vi "Set Quality Check Observables.vi"(8 "error in (no error)":errorcluster, 10 "Obsv to check":T1(array[cluster]), 11 "Schedule Block in":refnum<class "Schedule Block.lvclass">) -> (0 "error out":errorcluster, 3 "Schedule Block out":refnum<class "Schedule Block.lvclass">)   [LabVIEW 2020, in "TALOS.lvlib" / "Run Utilities.lvlib" / "Schedule Block.lvclass"]
uses:
  Schedule Block.lvclass
  Schedule Block.lvclass/Schedule Block.ctl
  Schedule/Schedule.lvclass
  Cell/Schedule Cell.lvclass
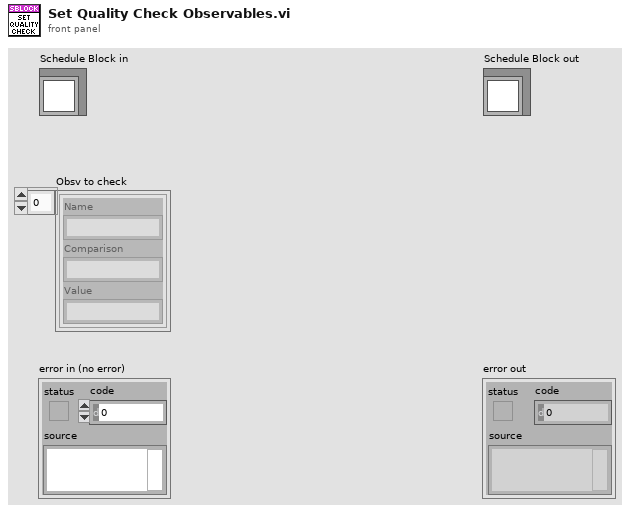
[diagram p1: front panel]
types:
  T1 = cluster{"Name":string, "Comparison":string, "Value":string}[]
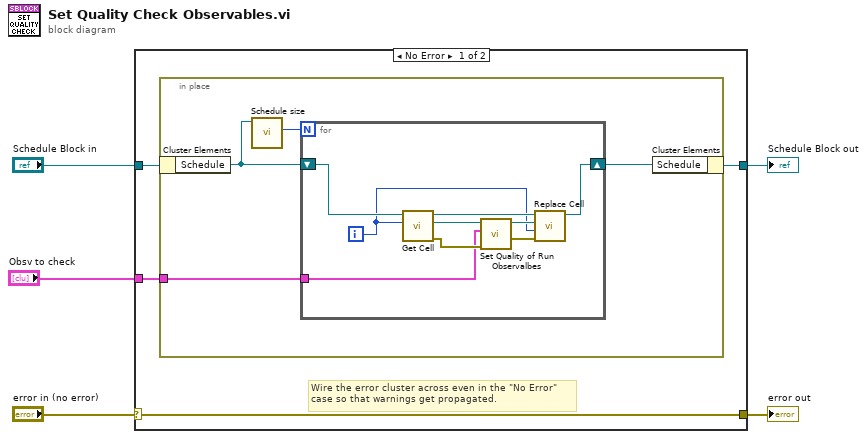
[diagram p0: block diagram]
diagram:
  n1 = case shown="No Error" "error in (no error)" {
    selector: "error in (no error)" -> [w9 w24]
    tunnel: [w9 w24] -> w4
    tunnel: [w7 w23] -> w2
    tunnel: "Schedule Block in" -> [w8 w23]
    tunnel: "Obsv to check" -> [w6 _]
    frame No Error {
      # "Wire the error cluster across even in the \"No Error\"\ncase so that warnings get propagated."
      n2 = in-place {
        in-place-border: w6 -> [w10]
        n3 = in-place-cluster #1(w8) -> ("Schedule"=w12:refnum<class "Schedule.lvclass">)
        n4 = call-dynamic "Schedule size.vi"("Schedule in"=w12) -> ("Size"=w13:i32)  [unwired: 8 in, 2 out]
        n5 = for {
          N: w13 -> [_]
          shift-right: [w20] -> w11
          shift-left: w12 -> [w22]
          tunnel: w10 -> [w14]
          i -> [w15]
          n6 = call-dynamic "Get Cell.vi"("index"=w15, "Schedule in"=w22) -> ("error out"=w18:errorcluster, "Schedule Cell"=w19:refnum<class "Schedule Cell.lvclass">, "Schedule out"=w21:refnum<class "Schedule.lvclass">)  [unwired: 7 in]
          n7 = call-dynamic "Set Quality of Run Observalbes.vi"("error in (no error)"=w18, "Obsv to check"=w14, "Schedule Cell in"=w19) -> ("error out"=w16:errorcluster, "Schedule Cell out"=w17:refnum<class "Schedule Cell.lvclass">)  [unwired: 7 in]
          n8 = call-dynamic "Replace Cell.vi"("error in (no error)"=w16, "Index"=w15, "Schedule Cell"=w17, "Schedule in"=w21) -> ("Schedule out"=w20:refnum<class "Schedule.lvclass">)  [unwired: 6 in, 1 out]
        }
        n9 = in-place-cluster #1("Schedule"=w11) -> (w7:refnum<class "Schedule Block.lvclass">)
      }
    }
    frame Error {
    }
  }
  "error out" <- w4
  "Schedule Block out" <- w2
